vi "Excel Add Printable Stat Lines.vi"(0 "CellsRefIn":refnum<k7>, 7 "RowIndex":i32, 11 "ErrorIn":errorcluster) -> (4 "CellsRefOut":refnum<k7>, 15 "ErrorOut":errorcluster)   [LabVIEW 2019]
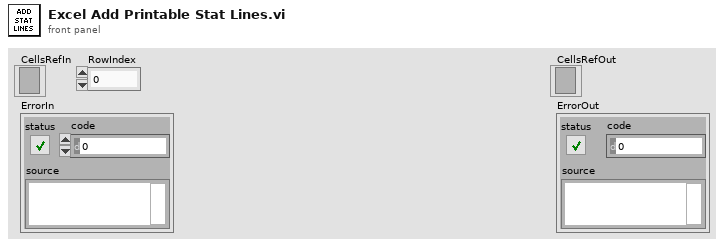
[diagram p1: front panel]
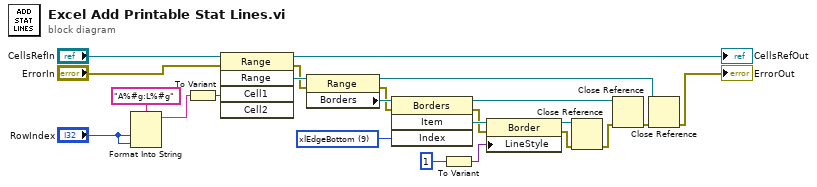
[diagram p0: block diagram]
diagram:
  w2 = 9 items=["xlInsideHorizontal"=12, "xlInsideVertical"=11, "xlDiagonalDown"=5, "xlDiagonalUp"=6, "xlEdgeBottom"=9, "xlEdgeLeft"=7, "xlEdgeRight"=10, "xlEdgeTop"=8] ("Index")
  n1 = Format Into String(format string="A%#g:L%#g", "RowIndex", "RowIndex") -> (resulting string=w1:string)  [unwired: 2 in, 1 out]
  n2 = To Variant(anything=w1) -> (Variant=w13:variant)
  n3 = invoke class="Range" method="Range"(reference="CellsRefIn", error in="ErrorIn", "Cell1"=w13) -> (reference out=→"CellsRefOut":refnum<k7>, error out=w16:errorcluster, "Range"=w18:refnum<k7>)  [unwired: 2 in, 2 out]
  n4 = property class="Range"(reference=w18, error in=w16) -> (reference out=w14:refnum<k7>, error out=w8:errorcluster, "Borders"=w10:refnum<k7>)
  n5 = invoke class="Borders" method="Item"(reference=w10, error in=w8, "Index"=w2) -> (reference out=w6:refnum<k7>, error out=w7:errorcluster, "Item"=w9:refnum<k7>)  [unwired: 1 in, 1 out]
  n6 = To Variant(anything=1 ("input 1")) -> (Variant=w12:variant)
  n7 = property class="Border"(reference=w9, error in=w7, "LineStyle"=w12) -> (reference out=w5:refnum<k7>, error out=w4:errorcluster)
  n8 = Close Reference(reference=w5, error in (no error)=w4) -> (error out=w3:errorcluster)
  n9 = Close Reference(reference=w6, error in (no error)=w3) -> (error out=w15:errorcluster)
  n10 = Close Reference(reference=w14, error in (no error)=w15) -> (error out=→"ErrorOut":errorcluster)
